vi "AT Flush A.vi"(8 "error in (no error)":errorcluster, 11 "Handle":i32) -> (0 "error out":errorcluster, 3 "Status":i32)   [LabVIEW 2019]
doc: "Flush\n\nReturn:\n I32 Status\n\nPrameters:\n I32 Handle\n\nThis function is used to flush out any remaining buffers that have been queued using the AT_QueueBuffer\nfunction. If this function is not called after an acquisition is complete then the remaining buffers will be used the next time an acquisition is started."
uses:
  atcoreA.dll
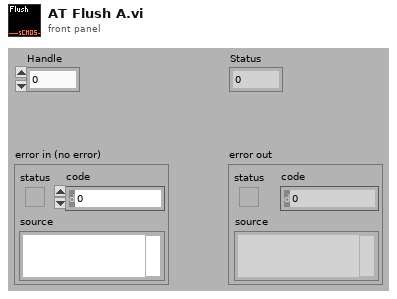
[diagram p1: front panel]
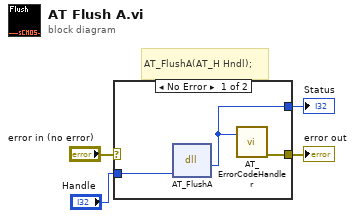
[diagram p0: block diagram]
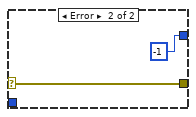
[diagram p2: hidden frame]
diagram:
  # "AT_FlushA(AT_H Hndl);"
  n1 = case shown="No Error" "error in (no error)" {
    selector: "error in (no error)" -> [_ w8]
    tunnel: [w6 w8] -> w3
    tunnel: "Handle" -> [w7 _]
    tunnel: [w5 -1] -> w1
    frame No Error {
      n2 = dll-call lib="atcoreA.dll" fn="AT_FlushA"("Handle"=w7) -> ("Status"=w5:i32)  [unwired: 4 in, 2 out]
      n3 = call "AT_ErrorCodeHandler.vi"("Error"=w5) -> ("error out"=w6:errorcluster)  [unwired: 6 in]
    }
    frame Error {
    }
  }
  "Status" <- w1
  "error out" <- w3
